vi "TAT_Com_PLC.vi"() -> ()   [LabVIEW 2017]
uses:
  <vilib>/NI/Modbus Library/API/Wrapper/Create TCP Master.vi
  Global/PLC_to_Auto.vi
  <vilib>/NI/Modbus Library/API/Master/Modbus Master.lvclass
  <vilib>/NI/Modbus Library/API/Wrapper/API Main.lvlib
panel:
  out "boolean out":bool[](array[boolean])
  out "Scanned Value D6000":string
  out "Write to PLC":bool[](array[boolean])
  out "error out":errorcluster
  out "Read set 1":u16[](array[numeric])
  out "PLC STATUS station 1":bool
  in  "error in":errorcluster
  in  "stop":bool
  # "STATION 1"
  # "CYCLE TIME\nAMBIENT TEMP\nBLINKER CURRENT OK\nTEMP SENSOR OK\nPART OK COUNT\nPART NOK COUNT\nFAULT BIT\nVARIENT\nHOUR\nMINUTE\nSECOND\nDAY\nMONTH\nYEAR\nSERIAL NUMBER\nShift\nAVM\nTS\nIV3"
  # "SCAN OK\nSCAN NG \nSoftware on Bit\nRQST FRM TCO REST SCN DT"
  # "BLINKER CURRENT OK\nTEMP SENSOR OK\nAVM OK\nIV3 CAMERA OK SIGNAL\nCYCLE COMPLETE\nCYCLE START (RUN CY)\nCYCLE STOP\nSCAN BYPASS\nRQS TO TCO READ SCN DTA"
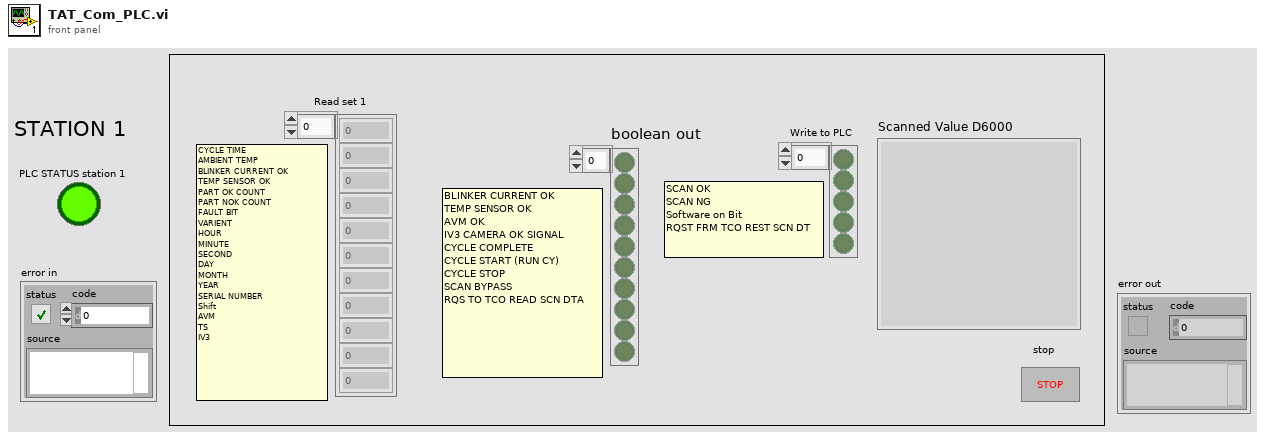
[diagram p1: front panel]
types:
  T1 = enum32{"invalid app kind", "Development System", "Run Time System", "Student Edition", "Embedded LabVIEW", "Evaluation", "Custom"}
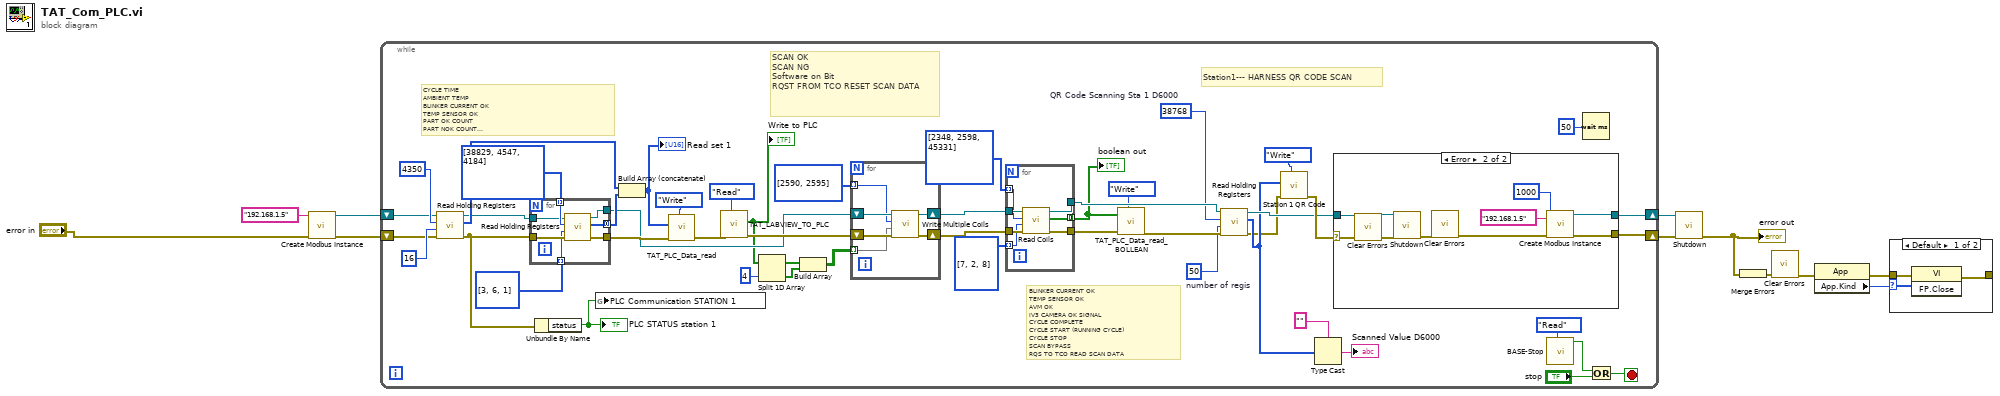
[diagram p0: block diagram]
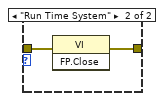
[diagram p3: hidden frame]
diagram:
  n1 = call-poly <vilib>:"Create Modbus Instance.vi"("error in"="error in", "address"="192.168.1.5") -> ("error out"=w6:errorcluster, "TCP master instance"=w5:refnum<class "Modbus Master.lvclass">)  [unwired: 8 in]
  n2 = while {
    shift-right: [w58] -> w10
    shift-left: w5 -> [w18]
    shift-right: [w57] -> w9
    shift-left: w6 -> [w19]
    stop <- w59 stop-if-true
    w38 = u16 50  # number of regis
    w39 = u16 38768  # QR Code Scanning Sta 1 D6000
    # "SCAN OK\nSCAN NG \nSoftware on Bit\nRQST FROM TCO RESET SCAN DATA"
    # "BLINKER CURRENT OK\nTEMP SENSOR OK\nAVM OK\nIV3 CAMERA OK SIGNAL\nCYCLE COMPLETE\nCYCLE START (RUNNING CYCLE)\nCYCLE STOP\nSCAN BYPASS\nRQS TO TCO READ SCAN DATA"
    # "Station1--- HARNESS QR CODE SCAN"
    # "CYCLE TIME\nAMBIENT TEMP\nBLINKER CURRENT OK\nTEMP SENSOR OK\nPART OK COUNT\nPART NOK COUNT\nFAULT BIT\nVARIENT\nHOUR\nMINUTE\nSECOND\nDAY\nMONTH\nYEAR\nSERIAL NUMBER\nShift\nAVM\nTS\nIV3 CAMERA"
    n3 = call-dynamic "Read Holding Registers.vi"("error in"=w19, "number of inputs"=u16 16, "starting address"=u16 4350 ("starting address 2"), "Modbus master in"=w18) -> ("error out"=w30:errorcluster, "register values"=w24:u16[], "Modbus master out"=w22:refnum<class "Modbus Master.lvclass">)  [unwired: 5 in]
    n4 = for {
      tunnel: u16[] [38829, 4547, 4184] ("starting address 2") -> [w90] mode=indexing
      tunnel: u16[] [3, 6, 1] ("number of inputs") -> [w89] mode=indexing
      tunnel: [w87] -> w23 mode=concatenating
      tunnel: w22 -> [w86]
      tunnel: [w85] -> w21
      tunnel: w30 -> [w91]
      tunnel: [w88] -> w26
      n5 = call-dynamic "Read Holding Registers.vi"("error in"=w91, "number of inputs"=w89, "starting address"=w90, "Modbus master in"=w86) -> ("error out"=w88:errorcluster, "register values"=w87:u16[], "Modbus master out"=w85:refnum<class "Modbus Master.lvclass">)  [unwired: 5 in]
    }
    n6 = Unbundle By Name(w30) -> ("status"=w47:bool)
    "PLC STATUS station 1" <- w47
    n7 = global write "PLC_to_Auto.vi" "PLC Communication STATION 1"(w47) -> ()
    n8 = Build Array (concatenate)(w24, w23) -> (w20:u16[])
    "Read set 1" <- w20
    n9 = call "TAT_PLC_Data_read.vi"("Enum"=enum16{"Read", "Write"}."Write", "error in (no error)"=w26, "Array"=w20) -> ("error out"=w25:errorcluster)  [unwired: 7 in, 1 out]
    n10 = call "TAT_LABVIEW_TO_PLC.vi"("Enum"=enum16{"Read", "Write"}."Read", "error in (no error)"=w25) -> ("error out"=w52:errorcluster, "Array 2"=w16:bool[])  [unwired: 8 in]
    "Write to PLC" <- w16
    n11 = Split 1D Array(array=w16, index=4) -> (first subarray=w15:bool[], second subarray=w14:bool[])
    n12 = Build Array(w15, w14) -> (w13:bool[][])
    n13 = for {
      tunnel: w13 -> [w83] mode=indexing
      shift-right: [w82] -> w49
      shift-left: w52 -> [w84]
      shift-right: [w81] -> w48
      shift-left: w21 -> [w80]
      tunnel: u16[] [2590, 2595] ("starting address") -> [w79] mode=indexing
      n14 = call-dynamic "Write Multiple Coils.vi"("error in"=w84, "coils to write"=w83, "starting address"=w79, "Modbus master in"=w80) -> ("error out"=w82:errorcluster, "Modbus master out"=w81:refnum<class "Modbus Master.lvclass">)  [unwired: 6 in]
    }
    n15 = for {
      tunnel: u16[] [7, 2, 8] ("number of inputs 2") -> [w64] mode=indexing
      tunnel: u16[] [2348, 2598, 45331] ("starting address 3") -> [w63] mode=indexing
      tunnel: w49 -> [w67]
      tunnel: [w62] -> w34
      tunnel: w48 -> [w66]
      tunnel: [w65] -> w41
      tunnel: [w61] -> w33 mode=concatenating
      n16 = call-dynamic "Read Coils.vi"("error in"=w67, "number of inputs"=w64, "starting address"=w63, "Modbus master in"=w66) -> ("error out"=w62:errorcluster, "coils"=w61:bool[], "Modbus master out"=w65:refnum<class "Modbus Master.lvclass">)  [unwired: 5 in]
    }
    "boolean out" <- w33
    n17 = call "TAT_PLC_Data_read_BOLLEAN.vi"("Enum"=enum16{"Read", "Write"}."Write", "error in (no error)"=w34, "Array"=w33) -> ("error out"=w42:errorcluster)  [unwired: 7 in, 1 out]
    n18 = call-dynamic "Read Holding Registers.vi"("error in"=w42, "number of inputs"=w38, "starting address"=w39, "Modbus master in"=w41) -> ("error out"=w31:errorcluster, "register values"=w32:u16[], "Modbus master out"=w40:refnum<class "Modbus Master.lvclass">)  [unwired: 5 in]
    n19 = call "Station 1 QR Code.vi"("Enum"=enum16{"Read", "Write"}."Write", "error in (no error)"=w31, "Array"=w32) -> ("error out"=w43:errorcluster)  [unwired: 7 in, 1 out]
    n20 = Type Cast(type="", x=w32) -> (*(type *) &x=→"Scanned Value D6000":string)
    n21 = case shown="Error" w43 {
      selector: w43 -> [w68 w78]
      tunnel: w40 -> [w69 w76]
      tunnel: [w69 w72] -> w58
      tunnel: [w68 w71] -> w57
      frame No Error {
      }
      frame Error {
        n22 = call <vilib>:"Clear Errors.vi"("error in (no error)"=w78) -> ("error out"=w77:errorcluster)  [unwired: 5 in, 1 out]
        n23 = call-dynamic "Shutdown.vi"("error in"=w77, "Modbus master in"=w76) -> ("error out"=w75:errorcluster)  [unwired: 9 in]
        n24 = call <vilib>:"Clear Errors.vi"("error in (no error)"=w75) -> ("error out"=w73:errorcluster)  [unwired: 5 in, 1 out]
        n25 = call-poly <vilib>:"Create Modbus Instance.vi"("error in"=w73, "connect timeout ms"=1000, "address"="192.168.1.5") -> ("error out"=w71:errorcluster, "TCP master instance"=w72:refnum<class "Modbus Master.lvclass">)  [unwired: 7 in]
      }
    }
    n26 = call "BASE-Stop.vi"("Enum"=enum16{"Read", "Write"}."Read") -> ("Stop"=w50:bool)  [unwired: 10 in]
    n27 = Wait (ms)(milliseconds to wait=u32 50) -> ()  [unwired: 1 out]
    n28 = Or(x=w50, y="stop") -> (x .or. y?=w59:bool)
  }
  n29 = call-dynamic "Shutdown.vi"("error in"=w9, "Modbus master in"=w10) -> ("error out"=w2:errorcluster)  [unwired: 9 in]
  "error out" <- w2
  n30 = Merge Errors(w2) -> (w1:errorcluster)
  n31 = call <vilib>:"Clear Errors.vi"("error in (no error)"=w1) -> ("error out"=w3:errorcluster)  [unwired: 5 in, 1 out]
  n32 = property class="App"(error in=w3) -> (error out=w7:errorcluster, "App.Kind"=w8:T1)  [unwired: 1 in, 1 out]
  n33 = case shown="Default" w8 {
    tunnel: w7 -> [w93 w95]
    tunnel: [w92 w94] -> _
    frame Default {
      n34 = invoke class="VI" method="FP.Close"(error in=w93) -> (error out=w92:errorcluster)  [unwired: 2 in, 2 out]
    }
    frame "Run Time System" {
      n35 = invoke class="VI" method="FP.Close"(error in=w95) -> (error out=w94:errorcluster)  [unwired: 2 in, 2 out]
    }
  }
